vi "Temperature plots.vi"(3 "lower limit":sgl=-20.0, 4 "upper limit":sgl=80.0, 5 "Temperatures":sgl[](array[numeric])) -> (0 "Sxx Chart":sgl(graph), 1 "Sxx histogram":T1(graph) caption="Temperature histogram")   [LabVIEW 2015, in "VIPM2.lvlib"]
uses:
  VIPM2.lvlib
  <vilib>/Analysis/NI_AALBase.lvlib
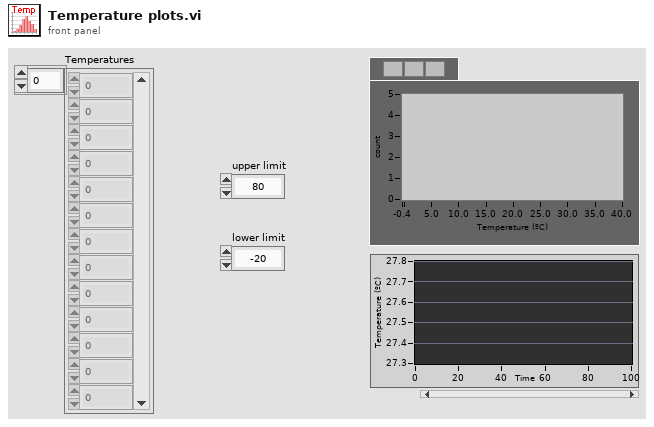
[diagram p1: front panel]
types:
  T1 = cluster{"X Values":dbl[], "Histogram: h(x)":i32[]}
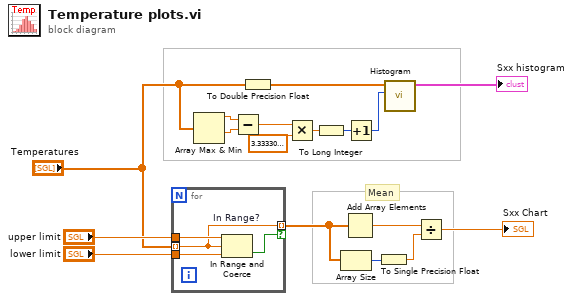
[diagram p0: block diagram]
diagram:
  # "Mean"
  n1 = for {
    tunnel: "Temperatures" -> [w19] mode=indexing
    tunnel: "upper limit" -> [w21]
    tunnel: "lower limit" -> [w20]
    tunnel: [w19] -> w15 mode=indexing if=w18
    n2 = In Range and Coerce "In Range?"(upper limit=w21, x=w19, lower limit=w20) -> (In Range?=w18:bool)  [unwired: 1 out]
  }
  n3 = Array Max & Min(array="Temperatures") -> (max value=w9:sgl, min value=w10:sgl)  [unwired: 2 out]
  n4 = Subtract(x=w9, y=w10) -> (x-y=w6:sgl)
  n5 = To Double Precision Float(number="Temperatures") -> (double precision float=w8:dbl[])
  n6 = Multiply(x=w6, y=sgl 3.3333 ("x")) -> (x*y=w4:sgl)
  n7 = To Long Integer(number=w4) -> (32bit integer=w3:i32)
  n8 = Array Size(array=w15) -> (size(s)=w14:i32)
  n9 = Add Array Elements(numeric array=w15) -> (sum=w12:sgl)
  n10 = Increment(x=w3) -> (x+1=w7:i32)
  n11 = To Single Precision Float(number=w14) -> (single precision float=w13:sgl)
  n12 = call <vilib>:"Histogram.vi"("intervals"=w7, "X"=w8) -> ("Histogram Graph"=→"Sxx histogram":T1)  [unwired: 6 in, 3 out]
  n13 = Divide(x=w12, y=w13) -> (x/y=→"Sxx Chart":sgl)
